vi "List Files.vi"(8 "error in":errorcluster, 11 "Cluster in":T1={"Running VI"=refnum, "Test VI"=refnum, "Q Ref"=refnum, "UE"=refnum, "Data"=variant, "Timeout"=-1, "ListBox[]"=[], "Source Path"=path "", "Delta Time"=0.0, "ExifInfo[]"=[], "ListIndex"=0, "counter"=0, "Format"=enum."Files Only", "total"=0, "Operation"=enum."Read Info", "Status"=""} {"ExifInfo[]"."New DateTime" format="%<%.3X>T"; "ExifInfo[]"."DateTimeOrginal" format="%<%.3X>T"}) -> (0 "error out":errorcluster, 3 "Cluster out":T1={"Running VI"=refnum, "Test VI"=refnum, "Q Ref"=refnum, "UE"=refnum, "Data"=variant, "Timeout"=-1, "ListBox[]"=[], "Source Path"=path "", "Delta Time"=0.0, "ExifInfo[]"=[], "ListIndex"=0, "counter"=0, "Format"=enum."Files Only", "total"=0, "Operation"=enum."Read Info", "Status"=""} {"ExifInfo[]"."New DateTime" format="%<%.3X>T"; "ExifInfo[]"."DateTimeOrginal" format="%<%.3X>T"})   [LabVIEW 2023, in "EXIF Modifier.lvlib"]
uses:
  EXIF Modifier.lvlib
  Controls/exif_consumer cluster.ctl
  Controls/exif_info cluster.ctl
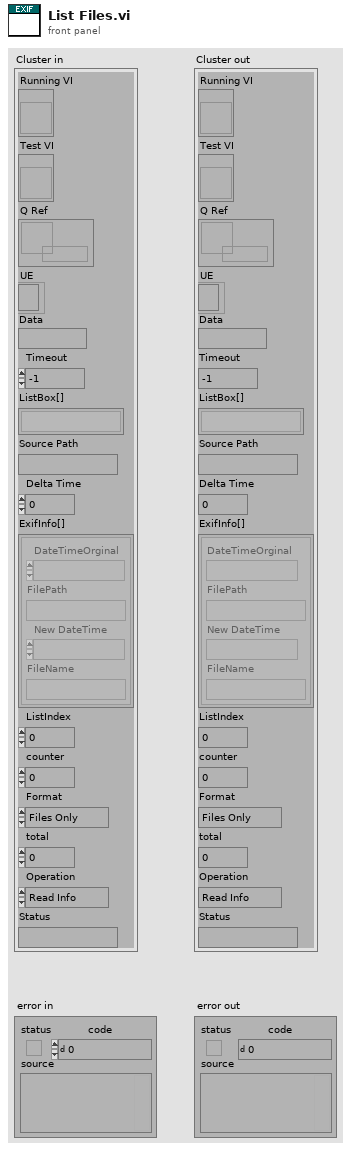
[diagram p1: front panel]
types:
  T1 = typedef "EXIF Modifier.lvlib/exif_consumer cluster.ctl" = cluster{"Running VI":refnum<vi>, "Test VI":refnum<vi>, "Q Ref":refnum<queue>, "UE":refnum<event-registration>, "Data":variant, "Timeout":i32, "ListBox[]":string[][], "Source Path":path, "Delta Time":dbl, "ExifInfo[]":T2[], "ListIndex":i32, "counter":i32, "Format":enum16{"Files Only", "Files Date", "All"}, "total":i32, "Operation":enum16{"Read Info", "Write Info"}, "Status":string}
  T2 = typedef "EXIF Modifier.lvlib/exif_info cluster.ctl" = cluster{"DateTimeOrginal":timestamp, "FilePath":path, "New DateTime":timestamp, "FileName":string}
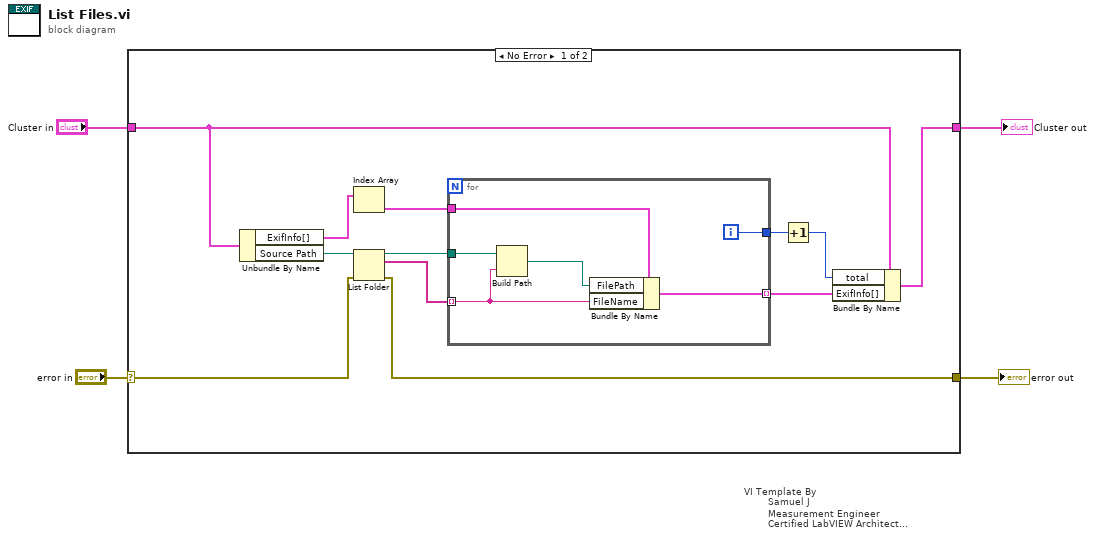
[diagram p0: block diagram]
diagram:
  n1 = case "VI Template By\n        Samuel J\n        Measurement Engineer\n        Certified LabVIEW Architect\n        Vestas Technology R&D Chennai" shown="No Error" "error in" {
    selector: "error in" -> [w7 w24]
    tunnel: [w6 w24] -> w3
    tunnel: [w9 w23] -> w1
    tunnel: "Cluster in" -> [w10 w23]
    frame No Error {
      n2 = Unbundle By Name(w10) -> ("ExifInfo[]"=w15:T2[], "Source Path"=w16:path)
      n3 = Index Array(array=w15) -> (element=w14:T2)  [unwired: 1 in]
      n4 = List Folder(path=w16, error in=w7) -> (path out=w12:path, filenames=w13:string[], error out=w6:errorcluster)  [unwired: 2 in, 1 out]
      n5 = for {
        tunnel: w14 -> [w22]
        tunnel: w13 -> [w20] mode=indexing
        tunnel: w12 -> [w21]
        tunnel: [w18] -> w11 mode=indexing
        tunnel: [w17] -> w8
        i -> [w17]
        n6 = Build Path(base path=w21, name or relative path=w20) -> (appended path=w19:path)
        n7 = Bundle By Name(cluster=w22, "FilePath"=w19, "FileName"=w20) -> (w18:T2)
      }
      n8 = Increment(x=w8) -> (x+1=w5:i32)
      n9 = Bundle By Name(cluster=w10, "total"=w5, "ExifInfo[]"=w11) -> (w9:T1)
    }
    frame Error {
    }
  }
  "error out" <- w3
  "Cluster out" <- w1
